vi "HistogramPlotProperties.vi"(4 "UCL":dbl, 5 "LCL":dbl, 6 "Zen Analytics in":refnum<class "Zen Analytics.lvclass">, 7 "Histogram Summary":refnum<vi>, 8 "error in (no error)":errorcluster, 9 "Plot Cluster Index out":cluster{"Plot Cluster":T1, i32}, 11 "HistogramValue":cluster{dbl[], dbl[]}[](graph)) -> (0 "error out":errorcluster)   [LabVIEW 2019, in "Zen Analytics.lvlib" / "Zen Analytics.lvclass"]
uses:
  Zen Analytics.lvclass
  Dependency/GraphReff.ctl
  <vilib>/ActorFramework/Message Enqueuer/Message Enqueuer.lvclass
  Dependency/AnalyticsDataToSM.ctl
  Dependency/Plot Cluster.ctl
types:
  T1 = typedef "Zen Analytics.lvlib/Zen Analytics.lvclass/Plot Cluster.ctl" = cluster{"Reduced 2D":dbl[][], "Start Index":i32, "No Of New Termnals":i32, "Top/Bottom":bool, "Values Inserted":i32, "Re-Initialised":bool, "Statistical params":string[][], "MeasurementInitializationData":cluster{"Measurement-ID":i32[], "Measurement Names":string[], "NominalValues":dbl[], "LSL":dbl[], "USL":dbl[], "LCL":dbl[], "UCL":dbl[]}, "MeasurementData":cluster{"Measurement ID":i32, "Measurement Name":string, "Nominal Values":dbl, "LSL":dbl, "USL":dbl, "LCL":dbl, "UCL":dbl}[], "ResultData2D":dbl[][], "PlotParameters":cluster{"Trend":cluster{"TrendPlotID":dbl, "PlotProperties":cluster{"FontName":string, "FontSize":dbl, "FontColor":string, "IsBold":bool, "IsItalic":bool, "PlotColor":string}}[], "Histogram":cluster{"HistogramPlotID":dbl, "PlotProperties":cluster{"FontName":string, "FontSize":dbl, "FontColor":string, "IsBold":bool, "IsItalic":bool, "PlotColor":string}}[], "BarPlot":cluster{"BarPlotID":dbl, "BarValuesID":dbl, "PlotProperties":cluster{"FontName":string, "FontSize":dbl, "IsBold":bool, "IsItalic":bool, "FontColor":string}, "Sectors":string[]}[], "PieChart":cluster{"PieChartID":dbl, "PieChartValueID":dbl, "PlotProperties":cluster{"FontName":string, "FontSize":dbl, "IsBold":bool, "IsItalic":bool, "FontColor":string}, "Sectors":string[]}[]}}
  T2 = cluster{"HistogramPlotID":dbl, "PlotProperties":cluster{"FontName":string, "FontSize":dbl, "FontColor":string, "IsBold":bool, "IsItalic":bool, "PlotColor":string}}[]
  T3 = cluster{"HistogramPlotID":dbl, "PlotProperties":cluster{"FontName":string, "FontSize":dbl, "FontColor":string, "IsBold":bool, "IsItalic":bool, "PlotColor":string}}
  T4 = typedef "Zen Analytics.lvlib/Zen Analytics.lvclass/AnalyticsDataToSM.ctl" = cluster{"Actor Info":cluster{"Analytics Enqueuer":refnum<class "Message Enqueuer.lvclass">, "This VI":refnum<vi>, "Module name":string}, "Statistical Info":string[][], "Graph Refference's":T5, "ErrorMessage":string}
  T5 = typedef "Zen Analytics.lvlib/Zen Analytics.lvclass/GraphReff.ctl" = cluster{"HistgramGraph-reff":refnum<vi>[], "BarGraph-reff":refnum<vi>[], "PieGraph-reff":refnum<vi>[], "Lable-reff":refnum<vi>[], "TrendGraph-reff":refnum<vi>[], "CpCpkTable":refnum<vi>}
  T6 = cluster{"FontName":string, "FontSize":dbl, "FontColor":string, "IsBold":bool, "IsItalic":bool, "PlotColor":string}
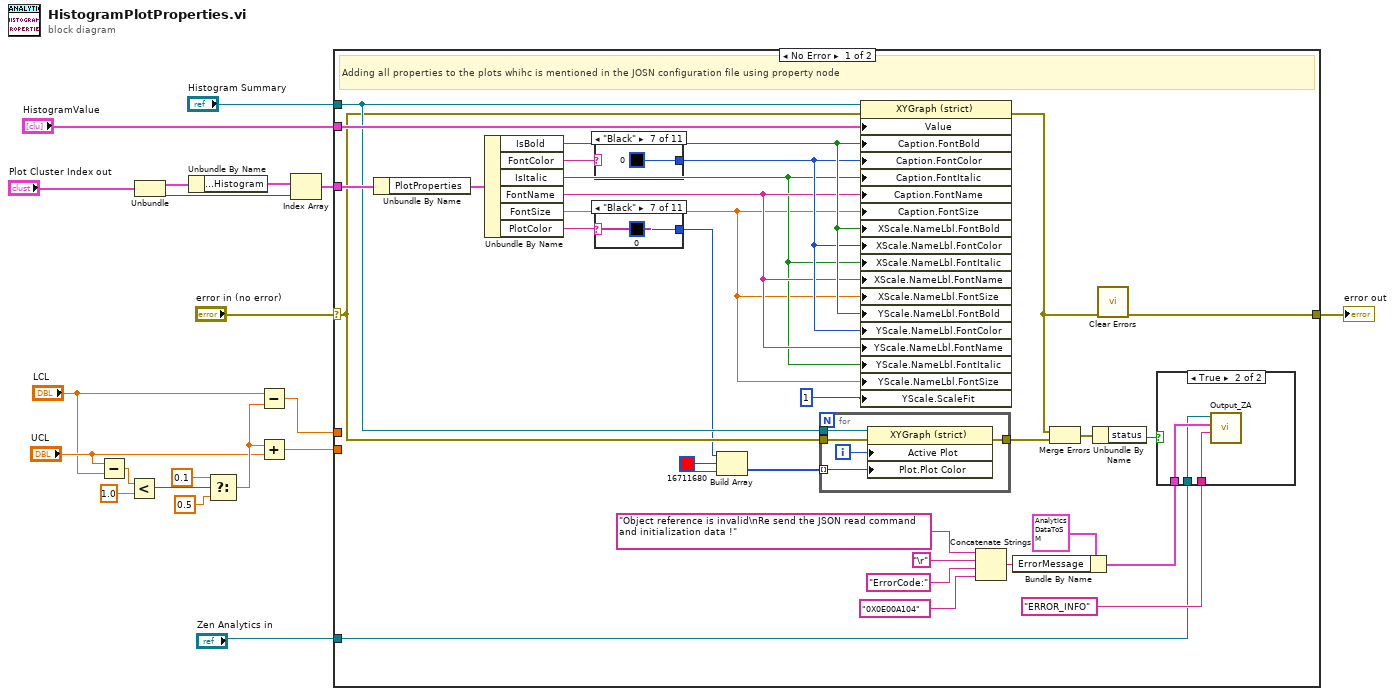
[diagram p0: block diagram]
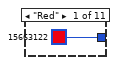
[diagram p3: hidden frame]
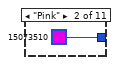
[diagram p4: hidden frame]
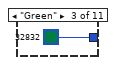
[diagram p5: hidden frame]
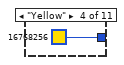
[diagram p6: hidden frame]
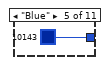
[diagram p7: hidden frame]
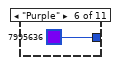
[diagram p8: hidden frame]
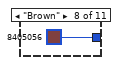
[diagram p9: hidden frame]
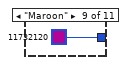
[diagram p10: hidden frame]
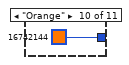
[diagram p11: hidden frame]
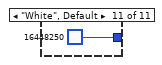
[diagram p12: hidden frame]
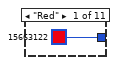
[diagram p13: hidden frame]
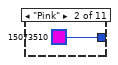
[diagram p14: hidden frame]
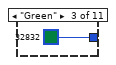
[diagram p15: hidden frame]
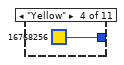
[diagram p16: hidden frame]
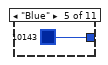
[diagram p17: hidden frame]
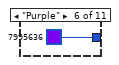
[diagram p18: hidden frame]
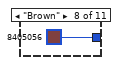
[diagram p19: hidden frame]
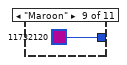
[diagram p20: hidden frame]
diagram:
  n1 = Subtract(x="UCL", y="LCL") -> (x-y=w10:dbl)
  n2 = Less?(x=w10, y=1.0) -> (x < y?=w8:bool)
  n3 = Unbundle("Plot Cluster Index out") -> ("Plot Cluster"=w15:T1, w17:i32)
  n4 = Unbundle By Name(w15) -> ("PlotParameters.Histogram"=w14:T2)
  n5 = Select(t=0.1, s=w8, f=0.5) -> (s? t:f=w5:dbl)
  n6 = Subtract(x="LCL", y=w5) -> (x-y=w19:dbl)
  n7 = Add(x=w5, y="UCL") -> (x+y=w18:dbl)
  n8 = Index Array(array=w14, index=w17) -> (element=w13:T3)
  n9 = case shown="No Error" "error in (no error)" {
    selector: "error in (no error)" -> [w26 w82]
    tunnel: w13 -> [w41 _]
    tunnel: "HistogramValue" -> [w42 _]
    tunnel: "Histogram Summary" -> [w27 _]
    tunnel: [w34 w81] -> w2
    tunnel: w19 -> [_ _]
    tunnel: w18 -> [_ _]
    tunnel: "Zen Analytics in" -> [w28 _]
    frame No Error {
      w22 = u32 16711680
      # "Adding all properties to the plots whihc is mentioned in the JOSN configuration file using property node"
      n10 = Unbundle By Name(w41) -> ("PlotProperties"=w49:T6)
      n11 = Unbundle By Name(w49) -> ("IsBold"=w48:bool, "FontColor"=w50:string, "IsItalic"=w45:bool, "FontName"=w46:string, "FontSize"=w44:dbl, "PlotColor"=w43:string)
      n12 = case shown="\"Black\"" w50 {
        tunnel: [u32 15663122 u32 15073510 u32 32832 u32 16768256 u32 10143 u32 7995636 u32 0 u32 8405056 u32 11732120 u32 16742144 u32 16448250] -> w47
        frame "Red" {
        }
        frame "Pink" {
        }
        frame "Green" {
        }
        frame "Yellow" {
        }
        frame "Blue" {
        }
        frame "Purple" {
        }
        frame "Black" {
        }
        frame "Brown" {
        }
        frame "Maroon" {
        }
        frame "Orange" {
        }
        frame "White", Default {
        }
      }
      n13 = case shown="\"Black\"" w43 {
        tunnel: [u32 15663122 u32 15073510 u32 32832 u32 16768256 u32 10143 u32 7995636 u32 0 u32 8405056 u32 11732120 u32 16742144 u32 16448250] -> w25
        frame "Red" {
        }
        frame "Pink" {
        }
        frame "Green" {
        }
        frame "Yellow" {
        }
        frame "Blue" {
        }
        frame "Purple" {
        }
        frame "Black" {
        }
        frame "Brown" {
        }
        frame "Maroon" {
        }
        frame "Orange" {
        }
        frame "White", Default {
        }
      }
      n14 = Build Array(w25, w22, w22) -> (w21:u32[])
      n15 = for {
        tunnel: w27 -> [w55]
        tunnel: w26 -> [w54]
        tunnel: [w52] -> w23
        tunnel: w21 -> [w51] mode=indexing
        i -> [w53]
        n16 = property on="Property Node" class="XYGraph (strict)"(reference=w55, error in=w54, "Active Plot"=w53, "Plot.Plot Color"=w51) -> (error out=w52:errorcluster)  [unwired: 1 out]
      }
      n17 = property on="Property Node" class="XYGraph (strict)"(reference=w27, error in=w26, "Value"=w42, "Caption.FontBold"=w48, "Caption.FontColor"=w47, "Caption.FontItalic"=w45, "Caption.FontName"=w46, "Caption.FontSize"=w44, "XScale.NameLbl.FontBold"=w48, "XScale.NameLbl.FontColor"=w47, "XScale.NameLbl.FontItalic"=w45, "XScale.NameLbl.FontName"=w46, "XScale.NameLbl.FontSize"=w44, "YScale.NameLbl.FontBold"=w48, "YScale.NameLbl.FontColor"=w47, "YScale.NameLbl.FontName"=w46, "YScale.NameLbl.FontItalic"=w45, "YScale.NameLbl.FontSize"=w44, "YScale.ScaleFit"=u8 1 ("Y Scale.Scale Fit")) -> (error out=w33:errorcluster)  [unwired: 1 out]
      n18 = Concatenate Strings("Object reference is invalid\nRe send the JSON read command and initialization data !" ("SolutionForError"), "\r", "ErrorCode:", "0X0E00A104" ("ErrorCode")) -> (w35:string)
      n19 = Bundle By Name(cluster=T4 {"Actor Info"={"Analytics Enqueuer"=refnum, "This VI"=refnum, "Module name"=""}, "Statistical Info"=[], "Graph Refference's"={"HistgramGraph-reff"=[], "BarGraph-reff"=[], "PieGraph-reff"=[], "Lable-reff"=[], "TrendGraph-reff"=[], "CpCpkTable"=refnum}, "ErrorMessage"=""} ("Analytics Information"), "ErrorMessage"=w35) -> (w30:T4)
      n20 = Merge Errors(w33, w23) -> (w24:errorcluster)
      n21 = Unbundle By Name(w24) -> ("status"=w32:bool)
      n22 = call <vilib>:"Clear Errors.vi"("error in (no error)"=w33) -> ("error out"=w34:errorcluster)  [unwired: 5 in, 1 out]
      n23 = case shown="True" w32 {
        tunnel: w30 -> [_ w58]
        tunnel: "ERROR_INFO" ("State") -> [_ w57]
        tunnel: w28 -> [_ w56]
        frame False {
        }
        frame True {
          n24 = call "Output_ZA.vi"("State"=w57, "Analytics Information"=w58, "Zen Analytics in"=w56) -> ()  [unwired: 7 in, 2 out]
        }
      }
    }
    frame Error {
      n25 = call <vilib>:"Clear Errors.vi"("error in (no error)"=w82) -> ("error out"=w81:errorcluster)  [unwired: 5 in, 1 out]
    }
  }
  "error out" <- w2
